vi "Send PreAddressed Return Msg.vi"(8 "error in (no error)":errorcluster, 11 "PreAddressedMsg in":refnum<class "PreAddressedMsg.lvclass">) -> (0 "error out":errorcluster, 3 "PreAddressedMsg out":refnum<class "PreAddressedMsg.lvclass">)   [LabVIEW 2017, in "AbstractMessages.lvlib" / "PreAddressedMsg.lvclass"]
uses:
  PreAddressedMsg.lvclass
  C:/Program Files (x86)/National Instruments/LabVIEW 2017/vi.lib/ActorFramework/Message/Message.lvclass
  PreAddressedMsg.lvclass/PreAddressedMsg.ctl
  <vilib>/ActorFramework/Message Enqueuer/Message Enqueuer.lvclass/Message Enqueuer.ctl
  <vilib>/ActorFramework/Message Priority Queue/Priority Enqueue.vi
  <vilib>/ActorFramework/Message Enqueuer/Message Enqueuer.lvclass
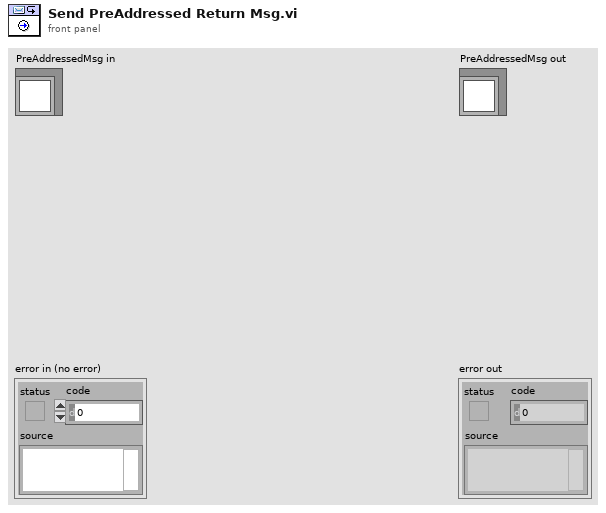
[diagram p1: front panel]
types:
  T1 = typedef "Actor Framework.lvlib/Message Enqueuer.lvclass/Message Priority.ctl" = enum16{"Low", "Normal", "High"}
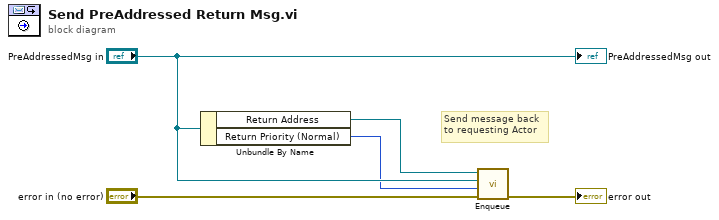
[diagram p0: block diagram]
diagram:
  # "Send message back\nto requesting Actor"
  n1 = Unbundle By Name("PreAddressedMsg in") -> ("Return Address"=w3:refnum<class "Message Enqueuer.lvclass">, "Return Priority (Normal)"=w1:T1)
  n2 = call <vilib>:"Enqueue.vi"("error in (no error)"="error in (no error)", "Message Priority (Normal)"=w1, "Message"="PreAddressedMsg in", "Message Enqueuer in"=w3) -> ("error out"=→"error out":errorcluster)  [unwired: 6 in, 1 out]
  "PreAddressedMsg out" <- "PreAddressedMsg in"
